vi "conversja na string.vi"(5 "max pwm skrecanie":i32, 7 "max obrót":i32, 8 "Z axis":i32, 9 "Y axis":i32, 10 "X axis":i32, 11 "max pwm przod":i32) -> (1 "obrot":i32, 2 "skrêt":i32, 3 "jazda":i32)   [LabVIEW 2015]
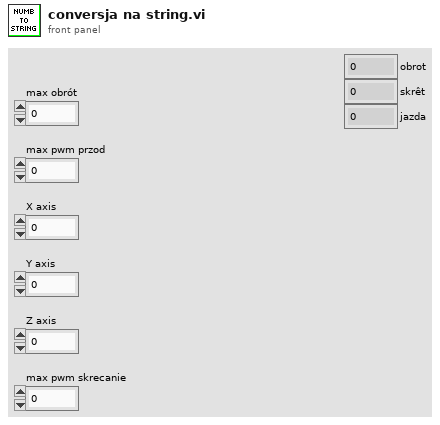
[diagram p1: front panel]
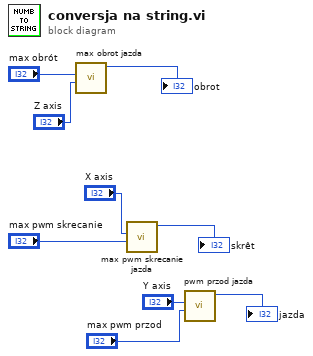
[diagram p0: block diagram]
diagram:
  n1 = call "max obrot jazda.vi"("Z axis"="Z axis", "max obrót"="max obrót") -> ("y"=→"obrot":i32)  [unwired: 9 in]
  n2 = call "max pwm skrecanie jazda.vi"("max pwm skrecanie"="max pwm skrecanie", "X axis"="X axis") -> ("y"=→"skrêt":i32)  [unwired: 9 in]
  n3 = call "pwm przod jazda.vi"("max pwm przod"="max pwm przod", "Y axis"="Y axis") -> ("Numeric"=→"jazda":i32)  [unwired: 9 in]
